vi "Open Port.vi"(8 "error in (no error)":errorcluster, 9 "targetCount":i32=1, 10 "VISA":refnum<visa-resource-name>, 11 "UART Actor in":refnum<class "UART Actor.lvclass">) -> (0 "error out":errorcluster, 3 "UART Actor out":refnum<class "UART Actor.lvclass">)   [LabVIEW 2020, in "UART Actor.lvlib" / "UART Actor.lvclass"]
uses:
  UART Actor.lvclass
  UART Actor.lvclass/UART Actor.ctl
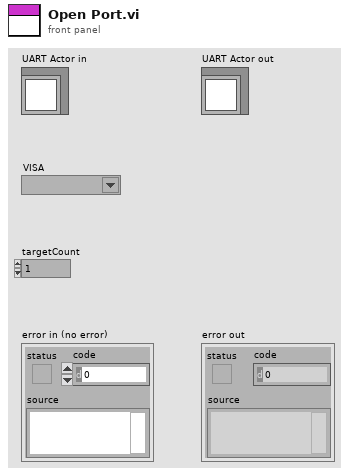
[diagram p1: front panel]
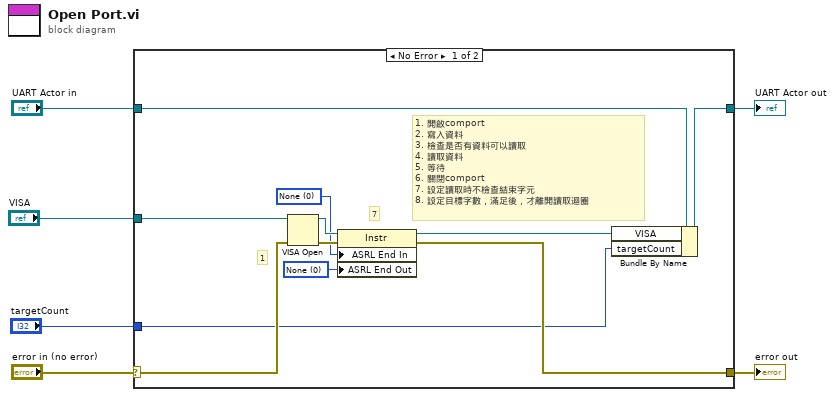
[diagram p0: block diagram]
diagram:
  n1 = case shown="No Error" "error in (no error)" {
    selector: "error in (no error)" -> [w12 w19]
    tunnel: [w11 w19] -> w5
    tunnel: [w10 w18] -> w3
    tunnel: "UART Actor in" -> [w17 w18]
    tunnel: "VISA" -> [w13 _]
    tunnel: "targetCount" -> [w8 _]
    frame No Error {
      w7 = u16 0 items=["None", "Last Bit", "TermChar", "Break"] ("Serial Settings:End Mode for Writes")
      w14 = u16 0 items=["None", "Last Bit", "TermChar"] ("Serial Settings:End Mode for Reads")
      # "1. 開啟comport\n2. 寫入資料\n3. 檢查是否有資料可以讀取\n4. 讀取資料\n5. 等待\n6. 關閉comport\n7. 設定讀取時不檢查結束字元\n8. 設定目標字數，滿足後，才離開讀取迴圈"
      # "7"
      # "1"
      n2 = VISA Open(error in (no error)=w12, VISA resource name=w13) -> (VISA resource name=w16:refnum<visa-resource-name>, error out=w15:errorcluster)  [unwired: 3 in]
      n3 = property class="Instr"(reference=w16, error in=w15, "ASRL End In"=w14, "ASRL End Out"=w7) -> (reference out=w9:refnum<visa-resource-name>, error out=w11:errorcluster)
      n4 = Bundle By Name(cluster=w17, "VISA"=w9, "targetCount"=w8) -> (w10:refnum<class "UART Actor.lvclass">)
    }
    frame Error {
    }
  }
  "error out" <- w5
  "UART Actor out" <- w3
